vi "DataColumnHead.vi"(8 "error in (no error)":errorcluster caption="错误输入（无错误）", 11 "TrendPlot 输入":refnum<class "TrendPlot.lvclass">) -> (0 "error out":errorcluster caption="错误输出", 2 "首行":string[](array[string]), 3 "TrendPlot 输出":refnum<class "TrendPlot.lvclass">)   [LabVIEW 2018, in "DataDisplay.lvlib" / "TrendPlot.lvclass"]
uses:
  TrendPlot.lvclass
  TrendPlot.lvclass/TrendPlot.ctl
  SubVI/DD_Parameter.vi
  DataDisplay.lvlib
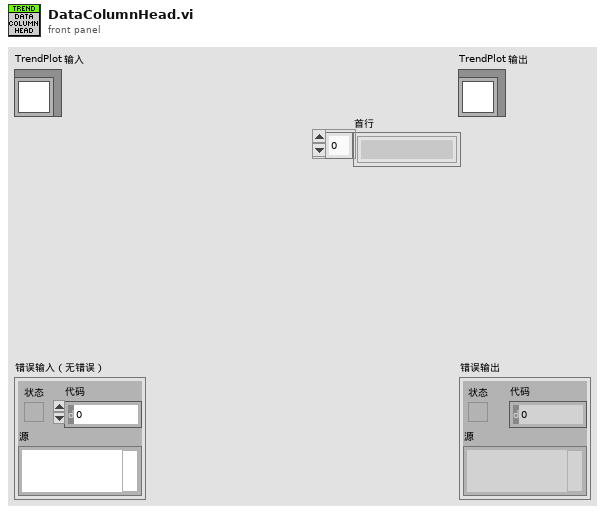
[diagram p1: front panel]
types:
  T1 = typedef "DataDisplay.lvlib/DD_ChannelInfo.ctl" = cluster{"名称":string, "单位":string, "数据类型":enum16{"Real", "Int"}, "趋势线":enum16{"N/A", "X", "Y"}}
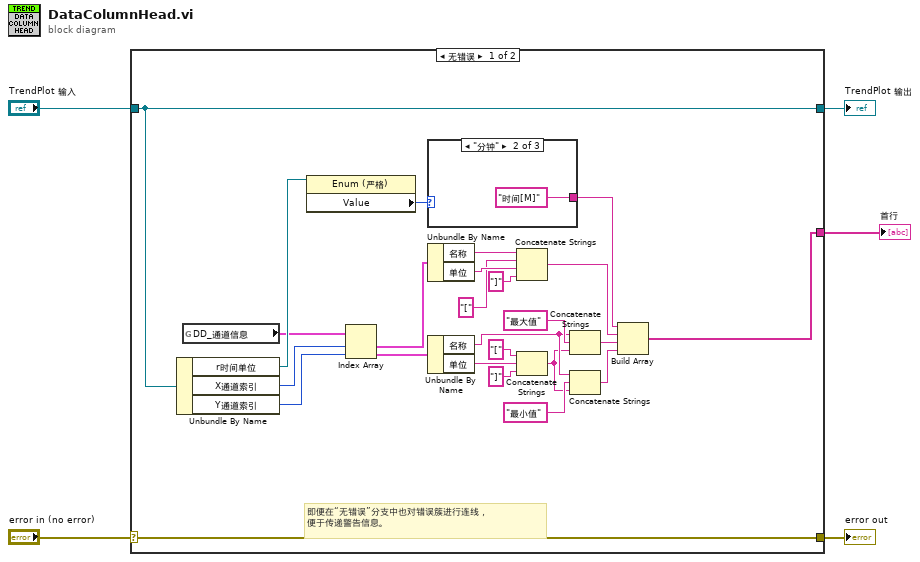
[diagram p0: block diagram]
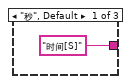
[diagram p2: hidden frame]
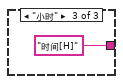
[diagram p3: hidden frame]
diagram:
  n1 = case shown="无错误" "error in (no error)" {
    selector: "error in (no error)" -> [w30 w35]
    tunnel: [w30 w35] -> w4
    tunnel: [w29 w34] -> w2
    tunnel: "TrendPlot 输入" -> [w29 w34]
    tunnel: [w6 _] -> w1
    frame No Error {
      # "即便在“无错误”分支中也对错误簇进行连线，\n便于传递警告信息。"
      n2 = Unbundle By Name(w29) -> ("r时间单位"=w28:refnum<vi>, "X通道索引"=w25:i32, "Y通道索引"=w24:i32)
      n3 = global read "DD_Parameter.vi" "DD_通道信息"() -> (w26:T1[])
      n4 = property class="Enum (严格)"(reference=w28) -> ("Value"=w27:enum16{"秒", "分钟", "小时"})  [unwired: 1 in, 2 out]
      n5 = Index Array(array=w26, index #1=w25, index #2=w24) -> (element #1=w23:T1, element #2=w18:T1)
      n6 = case shown="\"分钟\"" w27 {
        tunnel: ["时间[S]" "时间[M]" "时间[H]"] -> w10
        frame "秒", Default {
        }
        frame "分钟" {
        }
        frame "小时" {
        }
      }
      n7 = Unbundle By Name(w23) -> ("名称"=w22:string, "单位"=w21:string)
      n8 = Unbundle By Name(w18) -> ("名称"=w12:string, "单位"=w15:string)
      n9 = Concatenate Strings(w22, "[" ("字符串"), w21, "]" ("字符串")) -> (w9:string)
      n10 = Concatenate Strings("[" ("字符串"), w15, "]" ("字符串")) -> (w11:string)
      n11 = Concatenate Strings(w12, "最大值" ("字符串"), w11) -> (w8:string)
      n12 = Concatenate Strings(w12, "最小值" ("字符串"), w11) -> (w7:string)
      n13 = Build Array(w10, w9, w8, w7) -> (w6:string[])
    }
    frame Error {
    }
  }
  "error out" <- w4
  "TrendPlot 输出" <- w2
  "首行" <- w1
